vi "GetStimulusArrayValues.vi"(4 "tap train index":i32, 5 "time between onset index":i32, 6 "fraction of time between index":i32, 7 "Cluster":T1, 8 "time since beginning of run":i32) -> (0 "tap train index out":i32, 1 "time between onset index out":i32, 2 "fraction of time between index out":i32, 3 "stimulus settings":cluster{"outy3":sgl, "outy3":i32, "Value":i32})   [LabVIEW 2010]
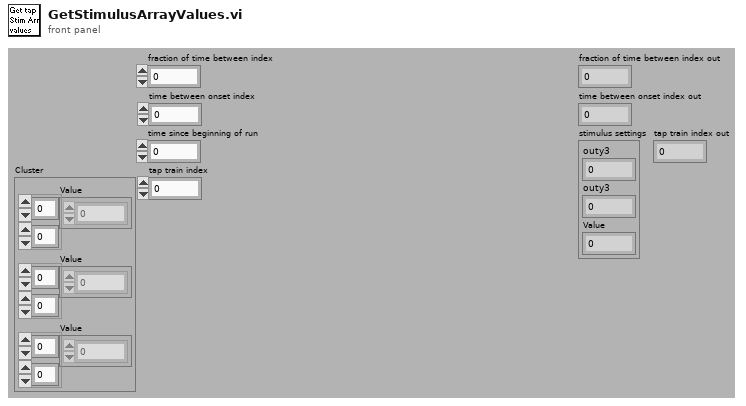
[diagram p1: front panel]
types:
  T1 = cluster{"Value":sgl[][], "Value":i32[][], "Value":i32[][]}
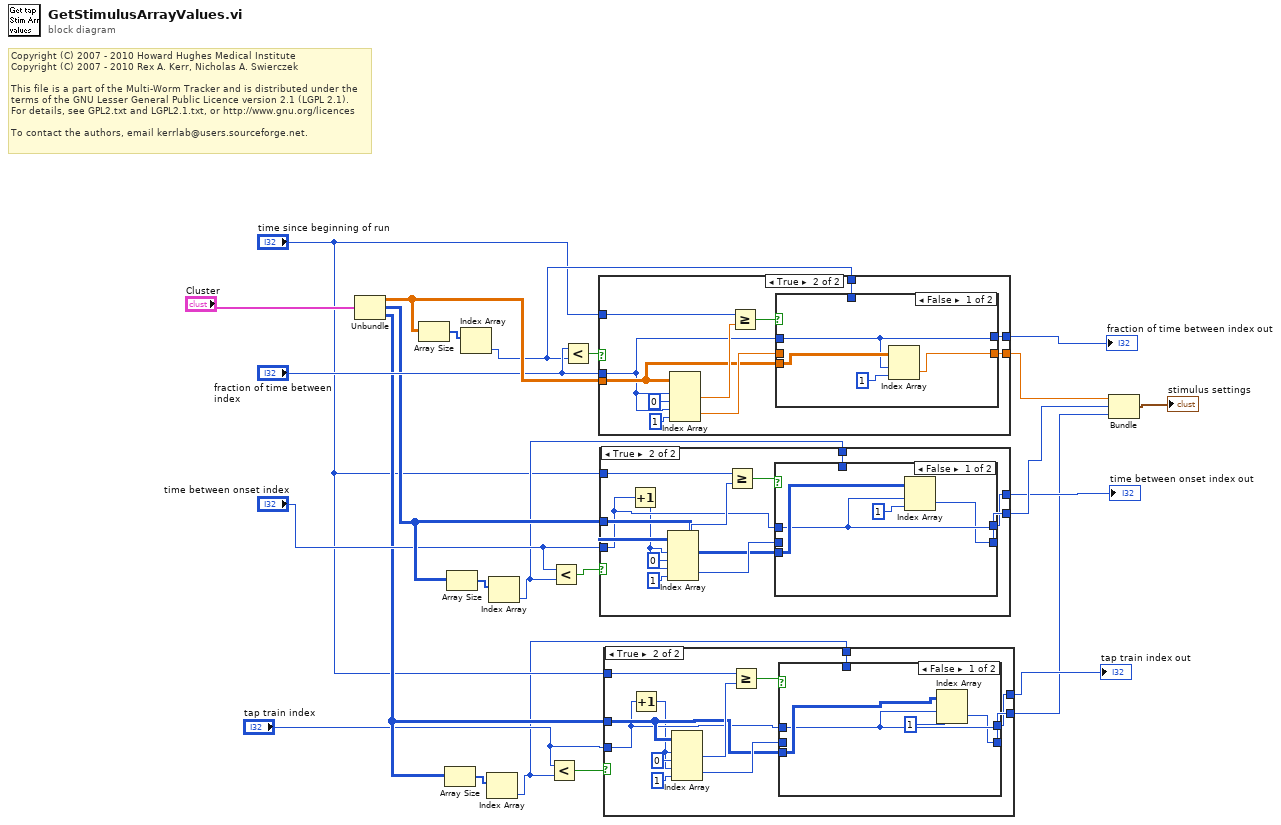
[diagram p0: block diagram]
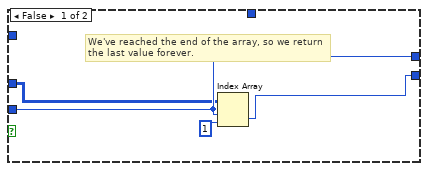
[diagram p2: hidden frame]
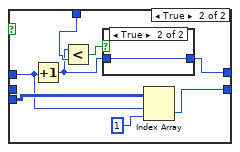
[diagram p3: hidden frame]
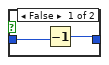
[diagram p4: hidden frame]
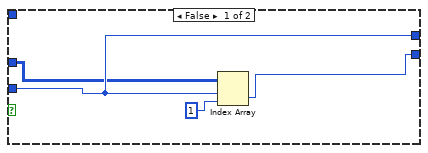
[diagram p5: hidden frame]
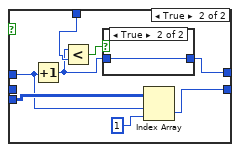
[diagram p6: hidden frame]
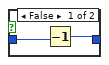
[diagram p7: hidden frame]
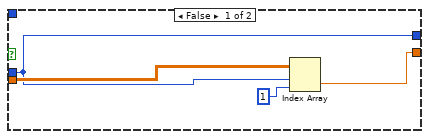
[diagram p8: hidden frame]
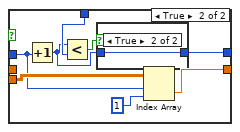
[diagram p9: hidden frame]
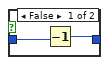
[diagram p10: hidden frame]
diagram:
  # "Copyright (C) 2007 - 2010 Howard Hughes Medical Institute\nCopyright (C) 2007 - 2010 Rex A. Kerr, Nicholas A. Swierczek\n \nThis file is a part of the Multi-Worm Tracker and is distributed under the\nterms of the GNU Lesser General Public Licence version 2.1 (LGPL 2.1).\nFor details, see GPL2.txt and LGPL2.1.txt, or http://www.gnu.org/licences\n \nTo contact the authors, email kerrlab@users.sourceforge.net."
  n1 = Unbundle("Cluster") -> ("Value"=w18:sgl[][], "Value"=w13:i32[][], "Value"=w6:i32[][])
  n2 = Array Size(array=w18) -> (size(s)=w17:i32[])
  n3 = Array Size(array=w6) -> (size(s)=w8:i32[])
  n4 = Array Size(array=w13) -> (size(s)=w14:i32[])
  n5 = Index Array(array=w17) -> (element=w11:i32)  [unwired: 1 in]
  n6 = Index Array(array=w8) -> (element=w3:i32)  [unwired: 1 in]
  n7 = Index Array(array=w14) -> (element=w10:i32)  [unwired: 1 in]
  n8 = Less?(x="tap train index", y=w3) -> (x < y?=w7:bool)
  n9 = Less?(x="time between onset index", y=w10) -> (x < y?=w15:bool)
  n10 = Less?(x="fraction of time between index", y=w11) -> (x < y?=w19:bool)
  n11 = case shown="True" w19 {
    tunnel: [w26 w35] -> w24
    tunnel: w18 -> [w27 w33]
    tunnel: "fraction of time between index" -> [w25 w32]
    tunnel: "time since beginning of run" -> [_ w31]
    tunnel: [w25 w30] -> w22
    tunnel: w11 -> [_ w29]
    frame False {
      n12 = Index Array(array=w27, index (row)=w25, index (col)=1 ("disabled index (col)")) -> (element=w26:sgl)
    }
    frame True {
      n13 = Index Array(array=w33, index (row) #1=w32, index (col) #1=0 ("disabled index (col)"), index (row) #2=w32, index (col) #2=1 ("disabled index (col)")) -> (element #1=w39:sgl, element #2=w34:sgl)
      n14 = Greater Or Equal?(x=w31, y=w39) -> (x >= y?=w36:bool)
      n15 = case shown="False" w36 {
        tunnel: [w41 w49] -> w35
        tunnel: w34 -> [_ _]
        tunnel: w32 -> [w40 w48]
        tunnel: [w40 w47] -> w30
        tunnel: w33 -> [w42 w51]
        tunnel: w29 -> [_ w46]
        frame False {
          n16 = Index Array(array=w42, index (row)=w40, index (col)=1 ("disabled index (col)")) -> (element=w41:sgl)
        }
        frame True {
          n17 = Increment(x=w48) -> (x+1=w44:i32)
          n18 = Less?(x=w44, y=w46) -> (x < y?=w45:bool)
          n19 = case shown="True" w45 {
            tunnel: [w52 w54] -> w47
            tunnel: w44 -> [w53 w54]
            frame False {
              n20 = Decrement(x=w53) -> (x-1=w52:i32)
            }
            frame True {
            }
          }
          n21 = Index Array(array=w51, index (row)=w48, index (col)=1 ("disabled index (col)")) -> (element=w49:sgl)
        }
      }
    }
  }
  "fraction of time between index out" <- w22
  n22 = case shown="True" w15 {
    tunnel: "time between onset index" -> [w57 w60]
    tunnel: [w55 w68] -> w23
    tunnel: "time since beginning of run" -> [_ w65]
    tunnel: w13 -> [w56 w63]
    tunnel: [w57 w62] -> w21
    tunnel: w10 -> [_ w61]
    frame False {
      n23 = Index Array(array=w56, index (row)=w57, index (col)=1 ("disabled index (col)")) -> (element=w55:i32)
    }
    frame True {
      n24 = Increment(x=w60) -> (x+1=w59:i32)
      n25 = Index Array(array=w63, index (row) #1=w59, index (col) #1=0 ("disabled index (col)"), index (row) #2=w59, index (col) #2=1 ("disabled index (col)")) -> (element #1=w66:i32, element #2=w64:i32)
      n26 = Greater Or Equal?(x=w65, y=w66) -> (x >= y?=w67:bool)
      n27 = case shown="False" w67 {
        tunnel: [w71 w80] -> w68
        tunnel: w64 -> [_ _]
        tunnel: w60 -> [w72 w79]
        tunnel: [w72 w76] -> w62
        tunnel: w63 -> [w73 w82]
        tunnel: w61 -> [_ w77]
        frame False {
          n28 = Index Array(array=w73, index (row)=w72, index (col)=1 ("disabled index (col)")) -> (element=w71:i32)
        }
        frame True {
          n29 = Increment(x=w79) -> (x+1=w75:i32)
          n30 = Less?(x=w75, y=w77) -> (x < y?=w78:bool)
          n31 = case shown="True" w78 {
            tunnel: [w83 w85] -> w76
            tunnel: w75 -> [w84 w85]
            frame False {
              n32 = Decrement(x=w84) -> (x-1=w83:i32)
            }
            frame True {
            }
          }
          n33 = Index Array(array=w82, index (row)=w79, index (col)=1 ("disabled index (col)")) -> (element=w80:i32)
        }
      }
    }
  }
  "time between onset index out" <- w21
  n34 = case shown="True" w7 {
    tunnel: "tap train index" -> [w88 w91]
    tunnel: [w86 w99] -> w1
    tunnel: "time since beginning of run" -> [_ w96]
    tunnel: w6 -> [w87 w94]
    tunnel: [w88 w93] -> w2
    tunnel: w3 -> [_ w92]
    frame False {
      # "We've reached the end of the array, so we return\nthe last value forever."
      n35 = Index Array(array=w87, index (row)=w88, index (col)=1 ("disabled index (col)")) -> (element=w86:i32)
    }
    frame True {
      n36 = Increment(x=w91) -> (x+1=w90:i32)
      n37 = Index Array(array=w94, index (row) #1=w90, index (col) #1=0 ("disabled index (col)"), index (row) #2=w90, index (col) #2=1 ("disabled index (col)")) -> (element #1=w97:i32, element #2=w95:i32)
      n38 = Greater Or Equal?(x=w96, y=w97) -> (x >= y?=w98:bool)
      n39 = case shown="False" w98 {
        tunnel: [w102 w111] -> w99
        tunnel: w95 -> [_ _]
        tunnel: w91 -> [w104 w110]
        tunnel: [w104 w107] -> w93
        tunnel: w94 -> [w105 w113]
        tunnel: w92 -> [_ w108]
        frame False {
          n40 = Index Array(array=w105, index (row)=w104, index (col)=1 ("disabled index (col)")) -> (element=w102:i32)
        }
        frame True {
          n41 = Increment(x=w110) -> (x+1=w106:i32)
          n42 = Less?(x=w106, y=w108) -> (x < y?=w109:bool)
          n43 = case shown="True" w109 {
            tunnel: [w114 w116] -> w107
            tunnel: w106 -> [w115 w116]
            frame False {
              n44 = Decrement(x=w115) -> (x-1=w114:i32)
            }
            frame True {
            }
          }
          n45 = Index Array(array=w113, index (row)=w110, index (col)=1 ("disabled index (col)")) -> (element=w111:i32)
        }
      }
    }
  }
  "tap train index out" <- w2
  n46 = Bundle("outy3"=w24, "outy3"=w23, "outy3"=w1) -> (→"stimulus settings":cluster{"outy3":sgl, "outy3":i32, "outy3":i32})  [unwired: 1 in]
